vi "Aux Scope Sync test.vi"() -> ()   [LabVIEW 2019]
uses:
  <vilib>/Platform/TimedLoop/XDataNode/timing_clust.ctl
  <vilib>/Platform/TimedLoop/XDataNode/nitl_modes.ctl
  <vilib>/Platform/TimedLoop/XDataNode/wakeup.ctl
  <vilib>/rvi/eio/common/nirviEmuTemplateMethod_errors.vi
  <vilib>/rvi/Emulation/niFpgaSctlEmulationGetInTimedLoop.vi
  <vilib>/rvi/Emulation/niFpgaEmulationReportErrorSimple.vi
  <vilib>/rvi/Emulation/niFpgaGetClockAttributes.vi
  <vilib>/rvi/Emulation/niFpgaCriticalErrorInLSC.vi
  <vilib>/eio/EIONode/EIONode.xnode
  <vilib>/platform/TimedLoop/XDataNode/XDataNode.xnode
  <vilib>/Platform/TimedLoop/XDataNode/XDNodeRunTimeDep.lvlib
panel:
  in  "stop":bool
  in  "Ring":i16(ring) items=["wait/start test", "forced clock"]
  in  "Single DIO/Bulk DIO":bool
  in  "Delay":i16(ring) items=["10 ticks", "50 ticks", "1 us", "1 ms", "100 ms", "1000 ms", "1 min"]
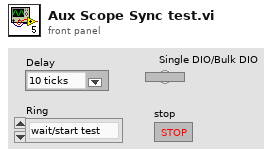
[diagram p1: front panel]
types:
  T1 = typedef "XDNodeRunTimeDep.lvlib/timing_clust.ctl" = cluster{"Expected End [f-1]":u64, "Actual End [f-1]":u64, "Finished Late? [f-1]":bool, "Expected End [i-1]":u64, "Actual End [i-1]":u64, "Finished Late? [i-1]":bool, "Expected Start [i]":u64, "Actual Start [i]":u64, "Expected Start [f]":u64, "Actual Start [f]":u64, "Source Name":string, "Structure Name":string, "Period":i64, "Deadline":i64, "Offset":i64, "Start":i64, "Priority":i32, "Timeout":i32, "Mode":T2, "Wakeup Reason":T3, "Error":errorcluster, "Source Type":string, "Secondary Source Type":string, "Global End Time":u64, "Global Start Time":u64, "Frame Duration":u64, "Iteration Duration":u64, "Assigned CPU":i32, "I/O Scan Engine Mode":u32}
  T2 = typedef "XDNodeRunTimeDep.lvlib/nitl_modes.ctl" = enum32{"No Change", "Process missed periods, maintain original phase", "Discard missed periods, maintain original phase", "Process missed periods, ignore original phase", "Discard missed periods, ignore original phase"}
  T3 = typedef "XDNodeRunTimeDep.lvlib/wakeup.ctl" = enum32{"Normal", "Aborted", "Asynchronous wakeup", "Timing source error", "Timed loop error", "Timeout"}
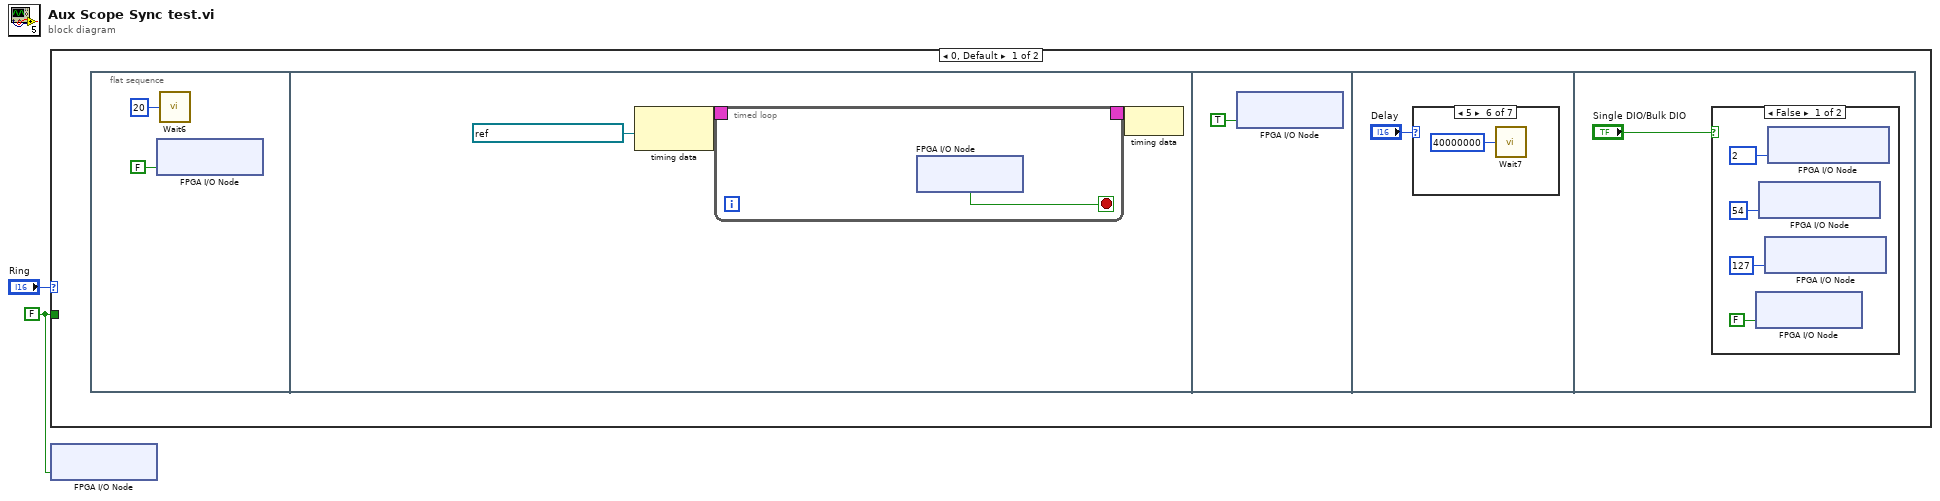
[diagram p0: block diagram]
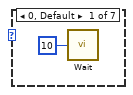
[diagram p2: hidden frame]
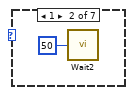
[diagram p3: hidden frame]
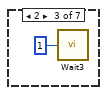
[diagram p4: hidden frame]
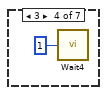
[diagram p5: hidden frame]
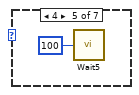
[diagram p6: hidden frame]
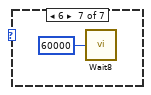
[diagram p7: hidden frame]
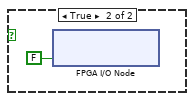
[diagram p8: hidden frame]
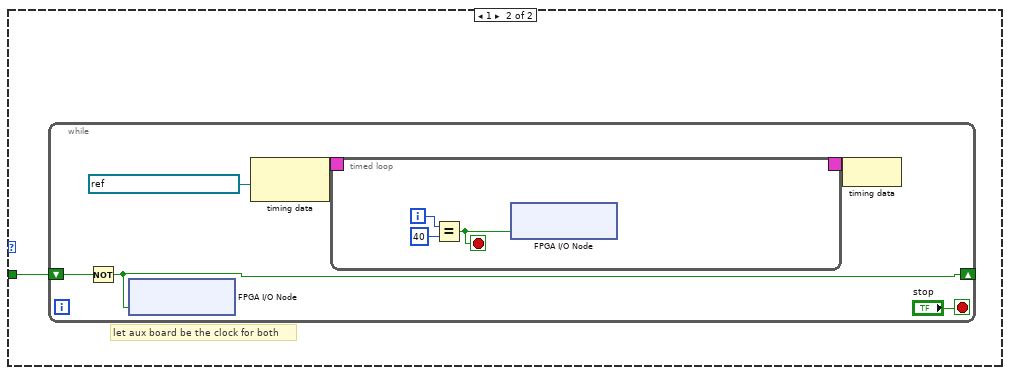
[diagram p9: hidden frame]
diagram:
  w1 = FALSE ("RMC/DIO47")
  n1 = case shown="0, Default" "Ring" {
    tunnel: w1 -> [_ w30]
    frame 0, Default {
      n2 = flat-sequence {
        frame #0 {
          n3 = xnode "FPGA I/O Node"("RMC/DIO32"=FALSE ("RMC/DIO47")) -> ()  [unwired: 1 in, 1 out]
          n4 = call "Wait6"("Count(mSec)"=u8 20) -> ()  [unwired: 1 out]
        }
        frame #1 {
          n5 = node-c288(refnum<k21> "40 MHz Onboard Clock" ("Source Name")) -> (w7:T1)
          n6 = timed-loop {
            timing: w7 -> [_]
            timing-out: [_] -> w6
            stop <- w8 stop-if-true
            n7 = xnode "FPGA I/O Node"() -> ("RMC/DIO47"=w8:bool)  [unwired: 1 in, 1 out]
          }
          n8 = node-c288(w6) -> ()
        }
        frame #2 {
          n9 = xnode "FPGA I/O Node"("RMC/DIO32"=TRUE ("RMC/DIO47")) -> ()  [unwired: 1 in, 1 out]
        }
        frame #3 {
          n10 = case shown="5" "Delay" {
            frame 0, Default {
              n11 = call "Wait"("Count(Ticks)"=u8 10) -> ()  [unwired: 1 out]
            }
            frame 1 {
              n12 = call "Wait2"("Count(Ticks)"=u8 50) -> ()  [unwired: 1 out]
            }
            frame 2 {
              n13 = call "Wait3"("Count(uSec)"=u8 1) -> ()  [unwired: 1 out]
            }
            frame 3 {
              n14 = call "Wait4"("Count(mSec)"=u32 1) -> ()  [unwired: 1 out]
            }
            frame 4 {
              n15 = call "Wait5"("Count(mSec)"=u32 100) -> ()  [unwired: 1 out]
            }
            frame 5 {
              n16 = call "Wait7"("Count(Ticks)"=u32 40000000) -> ()  [unwired: 1 out]
            }
            frame 6 {
              n17 = call "Wait8"("Count(mSec)"=u16 60000 ("Count(Ticks)")) -> ()  [unwired: 1 out]
            }
          }
        }
        frame #4 {
          n18 = case shown="False" "Single DIO/Bulk DIO" {
            frame False {
              n19 = xnode "FPGA I/O Node"("RMC/DIO32"=FALSE ("RMC/DIO47")) -> ()  [unwired: 1 in, 1 out]
              n20 = xnode "FPGA I/O Node"("RMC/DIO31:16"=u16 54) -> ()  [unwired: 1 in, 1 out]
              n21 = xnode "FPGA I/O Node"("RMC/DIO63:48"=u16 127 ("RMC/DIO79:64")) -> ()  [unwired: 1 in, 1 out]
              n22 = xnode "FPGA I/O Node"("RMC/DIO31:16"=u16 2) -> ()  [unwired: 1 in, 1 out]
            }
            frame True {
              n23 = xnode "FPGA I/O Node"("RMC/DIO32"=FALSE ("RMC/DIO47")) -> ()  [unwired: 1 in, 1 out]
            }
          }
        }
      }
    }
    frame 1 {
      # "let aux board be the clock for both"
      n24 = while {
        shift-right: [w32] -> _
        shift-left: w30 -> [w33]
        stop <- "stop" stop-if-true
        n25 = Not(x=w33) -> (.not. x?=w32:bool)
        n26 = xnode "FPGA I/O Node"("RMC/DIO83"=w32) -> ()  [unwired: 1 in, 1 out]
        n27 = node-c288(refnum<k21> "40 MHz Onboard Clock" ("Source Name")) -> (w36:T1)
        n28 = timed-loop {
          timing: w36 -> [_]
          timing-out: [_] -> w35
          i -> [w38]
          stop <- w37 stop-if-true
          n29 = Equal?(x=w38, y=u8 40) -> (x = y?=w37:bool)
          n30 = xnode "FPGA I/O Node"("RMC/DIO80"=w37) -> ()  [unwired: 1 in, 1 out]
        }
        n31 = node-c288(w35) -> ()
      }
    }
  }
  n32 = xnode "FPGA I/O Node"("RMC/DIO83"=w1) -> ()  [unwired: 1 in, 1 out]
